vi "widthCalculator.vi"(11 "Waveform Graph":dbl[](array[numeric])) -> (3 "Numeric":dbl)   [LabVIEW 2014]
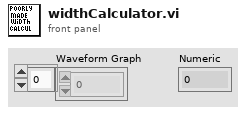
[diagram p1: front panel]
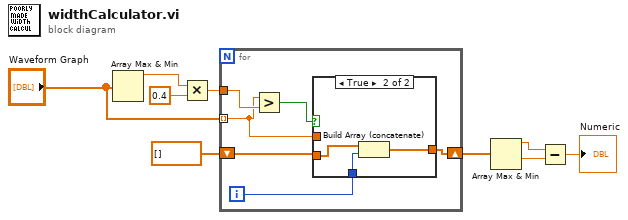
[diagram p0: block diagram]
diagram:
  n1 = Array Max & Min(array="Waveform Graph") -> (max value=w1:dbl)  [unwired: 3 out]
  n2 = Multiply(x=w1, y=0.4) -> (x*y=w4:dbl)
  n3 = for {
    tunnel: "Waveform Graph" -> [w13] mode=indexing
    tunnel: w4 -> [w15]
    shift-right: [w12] -> w6
    shift-left: dbl[] [] ("Waveform Graph 2") -> [w11]
    i -> [w10]
    n4 = Greater?(x=w13, y=w15) -> (0:w14:bool)
    n5 = case shown="True" w14 {
      tunnel: w11 -> [w16 w19]
      tunnel: w13 -> [_ _]
      tunnel: [w16 w18] -> w12
      tunnel: w10 -> [_ w17]
      frame False {
      }
      frame True {
        n6 = Build Array (concatenate)(w19, w17) -> (w18:dbl[])
      }
    }
  }
  n7 = Array Max & Min(array=w6) -> (max value=w7:dbl, min value=w8:dbl)  [unwired: 2 out]
  n8 = Subtract(x=w7, y=w8) -> (x-y=→"Numeric":dbl)
